vi "SentinelController v33.vi"() -> ()   [LabVIEW 2011] (continued)
                  n321 = property on="System UPH" class="Knob (strict)"("Scale.Minimum"=w3911) -> ()  [unwired: 2 in, 2 out]
                  n322 = property on="H1 UPH" class="Knob (strict)"("Scale.Minimum"=w3911) -> ()  [unwired: 2 in, 2 out]
                  n323 = property on="H2 UPH" class="Knob (strict)"("Scale.Minimum"=w3911) -> ()  [unwired: 2 in, 2 out]
                  n324 = property on="SysUtilMon" class="WFChart (strict)"("History Data"=cluster{dbl, dbl}[] []) -> ()  [unwired: 2 in, 2 out]
                  n325 = local write "H1 alarm"(w3929) -> ()
                  n326 = local write "H2 alarm"(w3929) -> ()
                  n327 = property on="YieldMon" class="WFChart (strict)"("History Data"=cluster{dbl, dbl, dbl, dbl}[] []) -> ()  [unwired: 2 in, 2 out]
                  n328 = local write "YieldMon"(w3906) -> ()
                  n329 = local write "SysUtilMon"(w3905) -> ()
                  n330 = local write "Sys utilization"(0.0) -> ()
                  n331 = local write "H2 alarm 2"(w3929) -> ()
                  n332 = local write "H1 alarm 2"(w3929) -> ()
                  n333 = local write "H2 nominal"(TRUE ("H1 nominal")) -> ()
                  n334 = local write "H1 nominal"(TRUE ("H1 nominal")) -> ()
                  n335 = local read "Lot number"() -> (w3903:string)
                  n336 = local write "Number of text alerts"(0.0 ("Number of Emails Alerts Sent")) -> ()
                  n337 = local write "Number of email alerts"(u32 0 ("Number of Emails Alerts Sent")) -> ()
                  n338 = local write "Tester loop counter hid"(u32 0 ("Tester loop counter")) -> ()
                  n339 = local write "H1 loop counter hid"(u32 0 ("H1 loop counter hid")) -> ()
                  n340 = local write "H2 loop counter hid"(u32 0 ("H2 loop counter hid")) -> ()
                  n341 = local write "H1 Ready with sites"(FALSE ("H1 Ready with sites")) -> ()
                  n342 = local write "H2 Ready with sites"(FALSE ("H1 Ready with sites")) -> ()
                  n343 = local write "GPIB Bus 0 traffic"(w3908) -> ()
                  n344 = local write "Notifications Lot Display"(w3903) -> ()
                  n345 = local write "GPIB bus 1 traffic"(w3908) -> ()
                  n346 = local write "GPIB bus 2 traffic"(w3908) -> ()
                }
              }
              n347 = case shown="True" w3812 {
                frame False {
                }
                frame True {
                  w3888 = FALSE
                  n348 = local read "H1 online"() -> (w3890:bool)
                  n349 = local read "H2 online"() -> (w3889:bool)
                  n350 = Equal?(x=w3890, y=w3888) -> (x = y?=w3892:bool)
                  n351 = Equal?(x=w3888, y=w3889) -> (x = y?=w3891:bool)
                  n352 = Or(x=w3892, y=w3891) -> (x .or. y?=w3887:bool)
                  n353 = case shown="True" w3887 {
                    frame False {
                    }
                    frame True {
                      n354 = local write "Optimize handler speed"(FALSE ("Optimize Handler Speed")) -> ()
                    }
                  }
                }
              }
              n355 = local read "Alert volume"() -> (w3823:u32)
              n356 = Equal To 0?(x=w3823) -> (x = 0?=w3825:bool)
              n357 = case shown="True" w3825 {
                frame False {
                }
                frame True {
                  n358 = local write "Audio On / Off"(FALSE ("Audio On/Off")) -> ()
                }
              }
            }
            n359 = case shown="True" FALSE {
              frame False {
              }
              frame True {
                n360 = while {
                  i -> [w1256]
                  stop <- w1269 stop-if-true
                  # "Play Audio Aert Loop"
                  n361 = local read "Ignore alarms until AFTER this many cycles"() -> (w1261:i32)
                  n362 = local read "H1 Device Count"() -> (w1266:u32)
                  n363 = local read "H2 Device Count"() -> (w1265:u32)
                  n364 = local read "Program Parallelism"() -> (w1263:u32)
                  n365 = local read "Run"() -> (w1258:bool)
                  n366 = local read "POWER"() -> (w1259:bool)
                  n367 = Add(x=w1266, y=w1265) -> (x+y=w1264:u32)
                  n368 = Wait (ms)(milliseconds to wait=u32 100) -> ()  [unwired: 1 out]
                  n369 = Divide(x=w1264, y=w1263) -> (x/y=w1262:dbl)
                  n370 = Greater?(x=w1256, y=50) -> (0:w1254:bool)
                  n371 = Greater?(x=w1262, y=w1261) -> (0:w1260:bool)
                  n372 = Compound Arithmetic op=AND(w1260, w1259, w1258, w1254) -> (w1257:bool)
                  n373 = case shown="True" w1257 {
                    frame False {
                    }
                    frame True {
                      n374 = local read "system statuts hid"() -> (w1273:T8)
                      n375 = case shown="\"H1AH2A\"" w1273 {
                        frame "H1NH2N", Default {
                          n376 = Wait (ms)(milliseconds to wait=u32 50) -> ()  [unwired: 1 out]
                        }
                        frame "H1NH2W" {
                          n377 = flat-sequence {
                            frame #0 {
                              n378 = local read "Audio On / Off"() -> (w1276:bool)
                              n379 = local read "H2 online"() -> (w1275:bool)
                              n380 = And(x=w1275, y=w1276) -> (x .and. y?=w1277:bool)
                              n381 = case shown="True" w1277 {
                                frame False {
                                }
                                frame True {
                                n382 = local read "Run"() -> (w1280:bool)
                                n383 = case shown="True" w1280 {
                                tunnel: [0.001 w1282] -> w1279
                                frame False {
                                }
                                frame True {
                                n384 = local read "Alert volume"() -> (w1282:u32)
                                }
                                }
                                n385 = call "PlayAlarm.vi"("wavefilename"="audio\\4_synth_warning.wav", "alertvolume"=w1279) -> ()  [unwired: 10 in]
                                }
                              }
                            }
                            frame #1 {
                              n386 = local read "Run"() -> (w1283:bool)
                              n387 = case shown="True" w1283 {
                                frame False {
                                }
                                frame True {
                                n388 = Wait (ms)(milliseconds to wait=u32 5000) -> ()  [unwired: 1 out]
                                }
                              }
                            }
                          }
                        }
                        frame "H1NH2A" {
                          n389 = flat-sequence {
                            frame #0 {
                              n390 = local read "Audio On / Off"() -> (w1287:bool)
                              n391 = local read "H2 online"() -> (w1286:bool)
                              n392 = And(x=w1286, y=w1287) -> (x .and. y?=w1285:bool)
                              n393 = case shown="True" w1285 {
                                frame False {
                                }
                                frame True {
                                n394 = local read "Run"() -> (w1290:bool)
                                n395 = case shown="True" w1290 {
                                tunnel: [0.001 w1292] -> w1289
                                frame False {
                                }
                                frame True {
                                n396 = local read "Alert volume"() -> (w1292:u32)
                                }
                                }
                                n397 = call "PlayAlarm.vi"("wavefilename"="audio\\bass_synth_alarm.wav", "alertvolume"=w1289) -> ()  [unwired: 10 in]
                                }
                              }
                            }
                            frame #1 {
                              n398 = local read "Run"() -> (w1293:bool)
                              n399 = case shown="True" w1293 {
                                frame False {
                                n400 = Wait (ms)(milliseconds to wait=u32 50) -> ()  [unwired: 1 out]
                                }
                                frame True {
                                n401 = Wait (ms)(milliseconds to wait=u32 5000) -> ()  [unwired: 1 out]
                                }
                              }
                            }
                          }
                        }
                        frame "H1WH2N" {
                          n402 = flat-sequence {
                            frame #0 {
                              n403 = local read "Audio On / Off"() -> (w1298:bool)
                              n404 = local read "H1 online"() -> (w1297:bool)
                              n405 = And(x=w1297, y=w1298) -> (x .and. y?=w1296:bool)
                              n406 = case shown="True" w1296 {
                                frame False {
                                }
                                frame True {
                                n407 = local read "Run"() -> (w1301:bool)
                                n408 = case shown="True" w1301 {
                                tunnel: [0.001 w1303] -> w1300
                                frame False {
                                }
                                frame True {
                                n409 = local read "Alert volume"() -> (w1303:u32)
                                }
                                }
                                n410 = call "PlayAlarm.vi"("wavefilename"="audio\\4_synth_warning.wav", "alertvolume"=w1300) -> ()  [unwired: 10 in]
                                }
                              }
                            }
                            frame #1 {
                              n411 = local read "Run"() -> (w1304:bool)
                              n412 = case shown="True" w1304 {
                                frame False {
                                n413 = Wait (ms)(milliseconds to wait=u32 50) -> ()  [unwired: 1 out]
                                }
                                frame True {
                                n414 = Wait (ms)(milliseconds to wait=u32 5000) -> ()  [unwired: 1 out]
                                }
                              }
                            }
                          }
                        }
                        frame "H1WH2W" {
                          n415 = flat-sequence {
                            frame #0 {
                              n416 = local read "Audio On / Off"() -> (w1310:bool)
                              n417 = local read "H1 online"() -> (w1307:bool)
                              n418 = local read "H2 online"() -> (w1309:bool)
                              n419 = Compound Arithmetic op=AND(w1307, w1309, w1310) -> (w1308:bool)
                              n420 = case shown="True" w1308 {
                                frame False {
                                }
                                frame True {
                                n421 = local read "Run"() -> (w1313:bool)
                                n422 = case shown="True" w1313 {
                                tunnel: [0.001 w1315] -> w1312
                                frame False {
                                }
                                frame True {
                                n423 = local read "Alert volume"() -> (w1315:u32)
                                }
                                }
                                n424 = call "PlayAlarm.vi"("wavefilename"="audio\\4_synth_warning.wav", "alertvolume"=w1312) -> ()  [unwired: 10 in]
                                }
                              }
                            }
                            frame #1 {
                              n425 = local read "Run"() -> (w1316:bool)
                              n426 = case shown="True" w1316 {
                                frame False {
                                n427 = Wait (ms)(milliseconds to wait=u32 50) -> ()  [unwired: 1 out]
                                }
                                frame True {
                                n428 = Wait (ms)(milliseconds to wait=u32 5000) -> ()  [unwired: 1 out]
                                }
                              }
                            }
                          }
                        }
                        frame "H1WH2A" {
                          n429 = flat-sequence {
                            frame #0 {
                              n430 = local read "Audio On / Off"() -> (w1322:bool)
                              n431 = local read "H1 online"() -> (w1320:bool)
                              n432 = local read "H2 online"() -> (w1321:bool)
                              n433 = Compound Arithmetic op=AND(w1320, w1321, w1322) -> (w1319:bool)
                              n434 = case shown="True" w1319 {
                                frame False {
                                }
                                frame True {
                                n435 = local read "Run"() -> (w1325:bool)
                                n436 = case shown="True" w1325 {
                                tunnel: [0.001 w1327] -> w1324
                                frame False {
                                }
                                frame True {
                                n437 = local read "Alert volume"() -> (w1327:u32)
                                }
                                }
                                n438 = call "PlayAlarm.vi"("wavefilename"="audio\\bass_synth_alarm.wav", "alertvolume"=w1324) -> ()  [unwired: 10 in]
                                }
                              }
                            }
                            frame #1 {
                              n439 = local read "Run"() -> (w1328:bool)
                              n440 = case shown="True" w1328 {
                                frame False {
                                n441 = Wait (ms)(milliseconds to wait=u32 50) -> ()  [unwired: 1 out]
                                }
                                frame True {
                                n442 = Wait (ms)(milliseconds to wait=u32 5000) -> ()  [unwired: 1 out]
                                }
                              }
                            }
                          }
                        }
                        frame "H1AH2N" {
                          n443 = flat-sequence {
                            frame #0 {
                              n444 = local read "Audio On / Off"() -> (w1333:bool)
                              n445 = local read "H1 online"() -> (w1331:bool)
                              n446 = And(x=w1331, y=w1333) -> (x .and. y?=w1332:bool)
                              n447 = case shown="True" w1332 {
                                frame False {
                                }
                                frame True {
                                n448 = local read "Run"() -> (w1336:bool)
                                n449 = case shown="True" w1336 {
                                tunnel: [0.001 w1338] -> w1335
                                frame False {
                                }
                                frame True {
                                n450 = local read "Alert volume"() -> (w1338:u32)
                                }
                                }
                                n451 = call "PlayAlarm.vi"("wavefilename"="audio\\bass_synth_alarm.wav", "alertvolume"=w1335) -> ()  [unwired: 10 in]
                                }
                              }
                            }
                            frame #1 {
                              n452 = local read "Run"() -> (w1339:bool)
                              n453 = case shown="True" w1339 {
                                frame False {
                                n454 = Wait (ms)(milliseconds to wait=u32 50) -> ()  [unwired: 1 out]
                                }
                                frame True {
                                n455 = Wait (ms)(milliseconds to wait=u32 5000) -> ()  [unwired: 1 out]
                                }
                              }
                            }
                          }
                        }
                        frame "H1AH2W" {
                          n456 = flat-sequence {
                            frame #0 {
                              n457 = local read "Audio On / Off"() -> (w1345:bool)
                              n458 = local read "H1 online"() -> (w1343:bool)
                              n459 = local read "H2 online"() -> (w1344:bool)
                              n460 = Compound Arithmetic op=AND(w1343, w1344, w1345) -> (w1342:bool)
                              n461 = case shown="True" w1342 {
                                frame False {
                                }
                                frame True {
                                n462 = local read "Run"() -> (w1348:bool)
                                n463 = case shown="True" w1348 {
                                tunnel: [0.001 w1350] -> w1347
                                frame False {
                                }
                                frame True {
                                n464 = local read "Alert volume"() -> (w1350:u32)
                                }
                                }
                                n465 = call "PlayAlarm.vi"("wavefilename"="audio\\bass_synth_alarm.wav", "alertvolume"=w1347) -> ()  [unwired: 10 in]
                                }
                              }
                            }
                            frame #1 {
                              n466 = local read "Run"() -> (w1351:bool)
                              n467 = case shown="True" w1351 {
                                frame False {
                                n468 = Wait (ms)(milliseconds to wait=u32 50) -> ()  [unwired: 1 out]
                                }
                                frame True {
                                n469 = Wait (ms)(milliseconds to wait=u32 5000) -> ()  [unwired: 1 out]
                                }
                              }
                            }
                          }
                        }
                        frame "H1AH2A" {
                          n470 = flat-sequence {
                            frame #0 {
                              n471 = local read "Audio On / Off"() -> (w1357:bool)
                              n472 = local read "H1 online"() -> (w1355:bool)
                              n473 = local read "H2 online"() -> (w1356:bool)
                              n474 = Compound Arithmetic op=AND(w1355, w1356, w1357) -> (w1354:bool)
                              n475 = case shown="True" w1354 {
                                frame False {
                                }
                                frame True {
                                n476 = local read "Run"() -> (w1360:bool)
                                n477 = case shown="True" w1360 {
                                tunnel: [0.001 w1362] -> w1359
                                frame False {
                                }
                                frame True {
                                n478 = local read "Alert volume"() -> (w1362:u32)
                                }
                                }
                                n479 = call "PlayAlarm.vi"("wavefilename"="audio\\bass_synth_alarm.wav", "alertvolume"=w1359) -> ()  [unwired: 10 in]
                                }
                              }
                            }
                            frame #1 {
                              n480 = local read "Run"() -> (w1363:bool)
                              n481 = case shown="True" w1363 {
                                frame False {
                                n482 = Wait (ms)(milliseconds to wait=u32 50) -> ()  [unwired: 1 out]
                                }
                                frame True {
                                n483 = Wait (ms)(milliseconds to wait=u32 5000) -> ()  [unwired: 1 out]
                                }
                              }
                            }
                          }
                        }
                      }
                    }
                  }
                  n484 = local read "Run"() -> (w1267:bool)
                  n485 = local read "POWER"() -> (w1270:bool)
                  n486 = Not(x=w1270) -> (.not. x?=w1272:bool)
                  n487 = Not(x=w1267) -> (.not. x?=w1271:bool)
                  n488 = Compound Arithmetic op=OR(w1272, w1271) -> (w1269:bool)
                }
              }
            }
            n489 = while {
              shift-right: [w3218] -> _
              shift-left: T8."H1NH2N" ("system statuts") -> [w3208]
              stop <- w3207 continue-if-true
              # "system status state machine:\n- writes data log whenever there is a change (if data loggin enabled)\n- issues email and text alerts is enabled (electronic notification of alarms)"
              n490 = local read "H1 parallelism"() -> (w3214:u32)
              n491 = local read "H1 Device Count"() -> (w3215:u32)
              n492 = local read "H2 Device Count"() -> (w3213:u32)
              n493 = local read "H2 parallelism"() -> (w3212:u32)
              n494 = local read "POWER"() -> (w3207:bool)
              n495 = Divide(x=w3213, y=w3212) -> (x/y=w3209:dbl)
              n496 = Divide(x=w3215, y=w3214) -> (x/y=w3210:dbl)
              n497 = local read "Ignore alarms until AFTER this many cycles"() -> (w3217:i32)
              n498 = Add(x=w3210, y=w3209) -> (x+y=w3211:dbl)
              n499 = Greater?(x=w3211, y=w3217) -> (0:w3216:bool)
              n500 = case shown="True" w3216 {
                tunnel: [w3220 w3223] -> w3218
                tunnel: w3208 -> [w3220 w3221]
                frame False {
                }
                frame True {
                  n501 = flat-sequence {
                    tunnel: [w3224] -> w3222
                    tunnel: w3221 -> [w3224]
                    tunnel: [w3321] -> w3223
                    tunnel: w3222 -> [w3319]
                    frame #0 {
                      # "Determine current state for System Status state-machine"
                      n502 = stacked-sequence {
                        frame #0 {
                          n503 = local read "H1 nominal 2"() -> (w3228:bool)
                          n504 = local read "H2 nominal 2"() -> (w3226:bool)
                          n505 = local read "H1 nominal"() -> (w3229:bool)
                          n506 = local read "H2 nominal"() -> (w3227:bool)
                          n507 = Compound Arithmetic op=AND(w3229, w3228, w3227, w3226) -> (w3225:bool)
                          n508 = case shown="True" w3225 {
                            frame False {
                            }
                            frame True {
                              n509 = local write "system statuts hid"(T8."H1NH2N" ("system statuts")) -> ()
                            }
                          }
                        }
                        frame #1 {
                          n510 = local read "H2 warning 2"() -> (w3233:bool)
                          n511 = local read "H2 warning"() -> (w3234:bool)
                          n512 = local read "H1 nominal 2"() -> (w3235:bool)
                          n513 = local read "H1 nominal"() -> (w3236:bool)
                          n514 = Or(x=w3234, y=w3233) -> (x .or. y?=w3232:bool)
                          n515 = Compound Arithmetic op=AND(w3236, w3235, w3232) -> (w3231:bool)
                          n516 = case shown="False" w3231 {
                            frame False {
                            }
                            frame True {
                              n517 = local write "system statuts hid"(T8."H1NH2W" ("system statuts")) -> ()
                            }
                          }
                        }
                        frame #2 {
                          n518 = local read "H1 nominal 2"() -> (w3243:bool)
                          n519 = local read "H1 nominal"() -> (w3244:bool)
                          n520 = local read "H2 alarm 2"() -> (w3241:bool)
                          n521 = local read "H2 alarm"() -> (w3242:bool)
                          n522 = Or(x=w3242, y=w3241) -> (x .or. y?=w3239:bool)
                          n523 = And(x=w3244, y=w3243) -> (x .and. y?=w3240:bool)
                          n524 = And(x=w3240, y=w3239) -> (x .and. y?=w3238:bool)
                          n525 = case shown="True" w3238 {
                            frame False {
                            }
                            frame True {
                              n526 = local write "system statuts hid"(T8."H1NH2A" ("system statuts")) -> ()
                            }
                          }
                        }
                        frame #3 {
                          n527 = local read "H1 alarm 2"() -> (w3254:bool)
                          n528 = local read "H1 alarm"() -> (w3255:bool)
                          n529 = local read "H2 nominal 2"() -> (w3257:bool)
                          n530 = local read "H1 warning 2"() -> (w3250:bool)
                          n531 = local read "H1 warning"() -> (w3251:bool)
                          n532 = local read "H2 nominal"() -> (w3256:bool)
                          n533 = Not(x=w3255) -> (.not. x?=w3253:bool)
                          n534 = Not(x=w3254) -> (.not. x?=w3252:bool)
                          n535 = Or(x=w3251, y=w3250) -> (x .or. y?=w3248:bool)
                          n536 = And(x=w3253, y=w3252) -> (x .and. y?=w3247:bool)
                          n537 = And(x=w3256, y=w3257) -> (x .and. y?=w3246:bool)
                          n538 = Compound Arithmetic op=AND(w3248, w3247, w3246) -> (w3249:bool)
                          n539 = case shown="True" w3249 {
                            frame False {
                            }
                            frame True {
                              n540 = local write "system statuts hid"(T8."H1WH2N" ("system statuts")) -> ()
                            }
                          }
                        }
                        frame #4 {
                          n541 = local read "H1 alarm 2"() -> (w3269:bool)
                          n542 = local read "H2 alarm 2"() -> (w3274:bool)
                          n543 = local read "H1 alarm"() -> (w3268:bool)
                          n544 = local read "H2 alarm"() -> (w3275:bool)
                          n545 = local read "H1 warning 2"() -> (w3265:bool)
                          n546 = local read "H2 warning 2"() -> (w3266:bool)
                          n547 = local read "H1 warning"() -> (w3264:bool)
                          n548 = local read "H2 warning"() -> (w3267:bool)
                          n549 = Not(x=w3268) -> (.not. x?=w3270:bool)
                          n550 = Not(x=w3269) -> (.not. x?=w3271:bool)
                          n551 = Not(x=w3275) -> (.not. x?=w3273:bool)
                          n552 = Not(x=w3274) -> (.not. x?=w3272:bool)
                          n553 = Or(x=w3264, y=w3265) -> (x .or. y?=w3262:bool)
                          n554 = Or(x=w3267, y=w3266) -> (x .or. y?=w3260:bool)
                          n555 = And(x=w3270, y=w3271) -> (x .and. y?=w3261:bool)
                          n556 = And(x=w3273, y=w3272) -> (x .and. y?=w3259:bool)
                          n557 = Compound Arithmetic op=AND(w3262, w3261, w3260, w3259) -> (w3263:bool)
                          n558 = case shown="True" w3263 {
                            frame False {
                            }
                            frame True {
                              n559 = local write "system statuts hid"(T8."H1WH2W" ("system statuts")) -> ()
                            }
                          }
                        }
                        frame #5 {
                          n560 = local read "H1 alarm 2"() -> (w3282:bool)
                          n561 = local read "H1 alarm"() -> (w3283:bool)
                          n562 = local read "H1 warning 2"() -> (w3285:bool)
                          n563 = local read "H1 warning"() -> (w3286:bool)
                          n564 = local read "H2 alarm 2"() -> (w3287:bool)
                          n565 = local read "H2 alarm"() -> (w3288:bool)
                          n566 = Not(x=w3283) -> (.not. x?=w3281:bool)
                          n567 = Not(x=w3282) -> (.not. x?=w3280:bool)
                          n568 = Or(x=w3286, y=w3285) -> (x .or. y?=w3279:bool)
                          n569 = Or(x=w3288, y=w3287) -> (x .or. y?=w3277:bool)
                          n570 = And(x=w3281, y=w3280) -> (x .and. y?=w3278:bool)
                          n571 = Compound Arithmetic op=AND(w3279, w3278, w3277) -> (w3284:bool)
                          n572 = case shown="True" w3284 {
                            frame False {
                            }
                            frame True {
                              n573 = local write "system statuts hid"(T8."H1WH2A" ("system statuts")) -> ()
                            }
                          }
                        }
                        frame #6 {
                          n574 = local read "H2 nominal 2"() -> (w3295:bool)
                          n575 = local read "H2 nominal"() -> (w3296:bool)
                          n576 = local read "H1 alarm 2"() -> (w3293:bool)
                          n577 = local read "H1 alarm"() -> (w3294:bool)
                          n578 = Or(x=w3294, y=w3293) -> (x .or. y?=w3291:bool)
                          n579 = And(x=w3296, y=w3295) -> (x .and. y?=w3290:bool)
                          n580 = And(x=w3291, y=w3290) -> (x .and. y?=w3292:bool)
                          n581 = case shown="True" w3292 {
                            frame False {
                            }
                            frame True {
                              n582 = local write "system statuts hid"(T8."H1AH2N" ("system statuts")) -> ()
                            }
                          }
                        }
                        frame #7 {
                          n583 = local read "H2 alarm 2"() -> (w3300:bool)
                          n584 = local read "H2 alarm"() -> (w3301:bool)
                          n585 = local read "H2 warning 2"() -> (w3306:bool)
                          n586 = local read "H2 warning"() -> (w3307:bool)
                          n587 = local read "H1 alarm 2"() -> (w3308:bool)
                          n588 = local read "H1 alarm"() -> (w3309:bool)
                          n589 = Not(x=w3301) -> (.not. x?=w3299:bool)
                          n590 = Not(x=w3300) -> (.not. x?=w3298:bool)
                          n591 = Or(x=w3309, y=w3308) -> (x .or. y?=w3304:bool)
                          n592 = Or(x=w3307, y=w3306) -> (x .or. y?=w3303:bool)
                          n593 = And(x=w3299, y=w3298) -> (x .and. y?=w3302:bool)
                          n594 = Compound Arithmetic op=AND(w3304, w3303, w3302) -> (w3305:bool)
                          n595 = case shown="True" w3305 {
                            frame False {
                            }
                            frame True {
                              n596 = local write "system statuts hid"(T8."H1AH2W" ("system statuts")) -> ()
                            }
                          }
                        }
                        frame #8 {
                          n597 = local read "H1 alarm 2"() -> (w3315:bool)
                          n598 = local read "H2 alarm 2"() -> (w3314:bool)
                          n599 = local read "H1 alarm"() -> (w3316:bool)
                          n600 = local read "H2 alarm"() -> (w3313:bool)
                          n601 = Or(x=w3316, y=w3315) -> (x .or. y?=w3311:bool)
                          n602 = Or(x=w3313, y=w3314) -> (x .or. y?=w3312:bool)
                          n603 = And(x=w3311, y=w3312) -> (x .and. y?=w3317:bool)
                          n604 = case shown="True" w3317 {
                            frame False {
                            }
                            frame True {
                              n605 = local write "system statuts hid"(T8."H1AH2A" ("system statuts")) -> ()
                            }
                          }
                        }
                      }
                    }
                    frame #1 {
                      n606 = local read "system statuts hid"() -> (w3321:T8)
                      n607 = Not Equal?(x=w3321, y=w3319) -> (x != y?=w3320:bool)
                      n608 = case shown="True" w3320 {
                        tunnel: w3321 -> [_ w3323]
                        frame False {
                        }
                        frame True {
                          n609 = local read "Enable data logging of all events"() -> (w3322:bool)
                          n610 = case shown="True" w3322 {
                            tunnel: w3323 -> [_ w3324]
                            frame False {
                            }
                            frame True {
                              n611 = stacked-sequence {
                                tunnel: w3324 -> [_ w3327 _ _ _]
                                frame #0 {
                                n612 = local read "Number of data log entries hid"() -> (w3326:u32)
                                n613 = Increment(x=w3326) -> (x+1=w3325:u32)
                                n614 = local write "Number of data log entries hid"(w3325) -> ()
                                }
                                frame #1 {
                                n615 = case shown="\"H1AH2A\"" w3327 {
                                frame "H1NH2N", Default {
                                w3334 = "\r\n"
                                n616 = local read "H1 online"() -> (w3351:bool)
                                n617 = local read "H2 online"() -> (w3352:bool)
                                n618 = local read "Number of data log entries hid"() -> (w3328:u32)
                                n619 = local read "H1 UPH warning limit hid"() -> (w3347:dbl)
                                n620 = local read "H2 UPH warning limit hid"() -> (w3349:dbl)
                                n621 = local read "YieldMon"() -> (w3332:cluster{i32, i32, i32, i32})
                                n622 = local read "H2  low yield warning"() -> (w3348:dbl)
                                n623 = local read "H1 low yield warning"() -> (w3346:dbl)
                                n624 = local read "H1 UPH"() -> (w3340:cluster{u32, u32})
                                n625 = local read "H2 UPH"() -> (w3338:cluster{u32, u32})
                                n626 = local read "YieldMon"() -> (w3330:cluster{i32, i32, i32, i32})
                                n627 = case shown="True" w3351 {
                                tunnel: ["H1 Off-Line" "H1 On-Line"] -> w3353
                                frame False {
                                }
                                frame True {
                                }
                                }
                                n628 = case shown="True" w3352 {
                                tunnel: ["H2 Off-Line" "H2 On-Line"] -> w3362
                                frame False {
                                }
                                frame True {
                                }
                                }
                                n629 = Unbundle(w3332) -> (w3331:i32)  [unwired: 3 out]
                                n630 = Unbundle(w3340) -> (w3339:u32)  [unwired: 1 out]
                                n631 = Unbundle(w3330) -> (w3329:i32)  [unwired: 3 out]
                                n632 = Unbundle(w3338) -> (w3337:u32)  [unwired: 1 out]
                                n633 = local read "Data log path and filename"() -> (w3336:path)
                                n634 = Number To Decimal String(number=w3346) -> (decimal integer string=w3355:string)  [unwired: 1 in]
                                n635 = Number To Decimal String(number=w3331) -> (decimal integer string=w3357:string)  [unwired: 1 in]
                                n636 = Number To Decimal String(number=w3347) -> (decimal integer string=w3359:string)  [unwired: 1 in]
                                n637 = Number To Decimal String(number=w3339) -> (decimal integer string=w3361:string)  [unwired: 1 in]
                                n638 = Number To Decimal String(number=w3348) -> (decimal integer string=w3364:string)  [unwired: 1 in]
                                n639 = Number To Decimal String(number=w3329) -> (decimal integer string=w3366:string)  [unwired: 1 in]
                                n640 = Number To Decimal String(number=w3349) -> (decimal integer string=w3368:string)  [unwired: 1 in]
                                n641 = Number To Decimal String(number=w3337) -> (decimal integer string=w3370:string)  [unwired: 1 in]
                                n642 = Number To Decimal String(number=w3328) -> (decimal integer string=w3333:string)  [unwired: 1 in]
                                n643 = Get Date/Time String(want seconds? (F)=TRUE) -> (date string=w3344:string, time string=w3345:string)  [unwired: 2 in]
                                n644 = Concatenate Strings(w3333, w3334, w3344, "   " ("string"), w3345, w3334, "H1 Nominal, H2 Nominal", w3334, w3353, w3334, "H1 Low Yield Warning Limit: ", w3355, ", H1 yield = ", w3357, w3334, "H1 Low UPH Warning Limit: ", w3359, ", H1 UPH = ", w3361, w3334, w3362, w3334, "H2 Low Yield Warning Limit: ", w3364, ", H2 yield = ", w3366, w3334, "H2 Low UPH Warning Limit: ", w3368, ", H2 UPH = ", w3370, w3334, w3334) -> (w3342:string)
                                n645 = call "SentinelDatalog.vi"("operation (0:open)"=T9."open", "String"=w3342, "data log path"=w3336) -> ()  [unwired: 8 in, 1 out]
                                }
                                frame "H1NH2W" {
                                w3380 = "\r\n"
                                n646 = local read "H1 online"() -> (w3398:bool)
                                n647 = local read "H2 online"() -> (w3399:bool)
                                n648 = local read "H1 UPH warning limit hid"() -> (w3394:dbl)
                                n649 = local read "H2 UPH warning limit hid"() -> (w3396:dbl)
                                n650 = local read "YieldMon"() -> (w3379:cluster{i32, i32, i32, i32})
                                n651 = local read "H2  low yield warning"() -> (w3395:dbl)
                                n652 = local read "H1 low yield warning"() -> (w3393:dbl)
                                n653 = local read "H1 UPH"() -> (w3387:cluster{u32, u32})
                                n654 = local read "H2 UPH"() -> (w3385:cluster{u32, u32})
                                n655 = local read "YieldMon"() -> (w3377:cluster{i32, i32, i32, i32})
                                n656 = local read "Number of data log entries hid"() -> (w3375:u32)
                                n657 = case shown="True" w3398 {
                                tunnel: ["H1 Off-Line" "H1 On-Line"] -> w3400
                                frame False {
                                }
                                frame True {
                                }
                                }
                                n658 = case shown="True" w3399 {
                                tunnel: ["H2 Off-Line" "H2 On-Line"] -> w3409
                                frame False {
                                }
                                frame True {
                                }
                                }
                                n659 = Unbundle(w3377) -> (w3376:i32)  [unwired: 3 out]
                                n660 = Unbundle(w3387) -> (w3386:u32)  [unwired: 1 out]
                                n661 = Unbundle(w3379) -> (w3378:i32)  [unwired: 3 out]
                                n662 = Unbundle(w3385) -> (w3384:u32)  [unwired: 1 out]
                                n663 = Number To Decimal String(number=w3393) -> (decimal integer string=w3402:string)  [unwired: 1 in]
                                n664 = Number To Decimal String(number=w3376) -> (decimal integer string=w3404:string)  [unwired: 1 in]
                                n665 = Number To Decimal String(number=w3394) -> (decimal integer string=w3406:string)  [unwired: 1 in]
                                n666 = Number To Decimal String(number=w3386) -> (decimal integer string=w3408:string)  [unwired: 1 in]
                                n667 = Number To Decimal String(number=w3395) -> (decimal integer string=w3411:string)  [unwired: 1 in]
                                n668 = Number To Decimal String(number=w3378) -> (decimal integer string=w3413:string)  [unwired: 1 in]
                                n669 = Number To Decimal String(number=w3396) -> (decimal integer string=w3415:string)  [unwired: 1 in]
                                n670 = Number To Decimal String(number=w3384) -> (decimal integer string=w3417:string)  [unwired: 1 in]
                                n671 = Number To Decimal String(number=w3375) -> (decimal integer string=w3381:string)  [unwired: 1 in]
                                n672 = local read "Data log path and filename"() -> (w3383:path)
                                n673 = Get Date/Time String(want seconds? (F)=TRUE) -> (date string=w3391:string, time string=w3392:string)  [unwired: 2 in]
                                n674 = Concatenate Strings(w3381, w3380, w3391, "   " ("string"), w3392, w3380, "H1 Nominal, H2 Warning", w3380, w3400, w3380, "H1 Low Yield Warning Limit: ", w3402, ", H1 yield = ", w3404, w3380, "H1 Low UPH Warning Limit: ", w3406, ", H1 UPH = ", w3408, w3380, w3409, w3380, "H2 Low Yield Warning Limit: ", w3411, ", H2 yield = ", w3413, w3380, "H2 Low UPH Warning Limit: ", w3415, ", H2 UPH = ", w3417, w3380, w3380) -> (w3389:string)
                                n675 = call "SentinelDatalog.vi"("operation (0:open)"=T9."open", "String"=w3389, "data log path"=w3383) -> ()  [unwired: 8 in, 1 out]
                                }
                                frame "H1NH2A" {
                                w3428 = "\r\n"
                                n676 = local read "H1 online"() -> (w3445:bool)
                                n677 = local read "H2 online"() -> (w3446:bool)
                                n678 = local read "Number of data log entries hid"() -> (w3422:u32)
                                n679 = local read "H1 UPH warning limit hid"() -> (w3441:dbl)
                                n680 = local read "H1 low yield warning"() -> (w3440:dbl)
                                n681 = local read "H2 UPH alarm limit hid"() -> (w3443:dbl)
                                n682 = local read "YieldMon"() -> (w3426:cluster{i32, i32, i32, i32})
                                n683 = local read "H1 UPH"() -> (w3434:cluster{u32, u32})
                                n684 = local read "H2 low yield alarm"() -> (w3442:dbl)
                                n685 = local read "H2 UPH"() -> (w3433:cluster{u32, u32})
                                n686 = local read "YieldMon"() -> (w3424:cluster{i32, i32, i32, i32})
                                n687 = case shown="True" w3445 {
                                tunnel: ["H1 Off-Line" "H1 On-Line"] -> w3447
                                frame False {
                                }
                                frame True {
                                }
                                }
                                n688 = case shown="True" w3446 {
                                tunnel: ["H2 Off-Line" "H2 On-Line"] -> w3456
                                frame False {
                                }
                                frame True {
                                }
                                }
                                n689 = Number To Decimal String(number=w3422) -> (decimal integer string=w3427:string)  [unwired: 1 in]
                                n690 = Unbundle(w3426) -> (w3425:i32)  [unwired: 3 out]
                                n691 = Unbundle(w3434) -> (w3431:u32)  [unwired: 1 out]
                                n692 = Unbundle(w3424) -> (w3423:i32)  [unwired: 3 out]
                                n693 = Unbundle(w3433) -> (w3432:u32)  [unwired: 1 out]
                                n694 = Number To Decimal String(number=w3440) -> (decimal integer string=w3449:string)  [unwired: 1 in]
                                n695 = Number To Decimal String(number=w3425) -> (decimal integer string=w3451:string)  [unwired: 1 in]
                                n696 = Number To Decimal String(number=w3441) -> (decimal integer string=w3453:string)  [unwired: 1 in]
                                n697 = Number To Decimal String(number=w3431) -> (decimal integer string=w3455:string)  [unwired: 1 in]
                                n698 = Number To Decimal String(number=w3442) -> (decimal integer string=w3458:string)  [unwired: 1 in]
                                n699 = Number To Decimal String(number=w3423) -> (decimal integer string=w3460:string)  [unwired: 1 in]
                                n700 = Number To Decimal String(number=w3443) -> (decimal integer string=w3462:string)  [unwired: 1 in]
                                n701 = Number To Decimal String(number=w3432) -> (decimal integer string=w3464:string)  [unwired: 1 in]
                                n702 = local read "Data log path and filename"() -> (w3430:path)
                                n703 = Get Date/Time String(want seconds? (F)=TRUE) -> (date string=w3438:string, time string=w3439:string)  [unwired: 2 in]
                                n704 = Concatenate Strings(w3427, w3428, w3438, "   " ("string"), w3439, w3428, "H1 Nominal, H2 Alarming", w3428, w3447, w3428, "H1 Low Yield Warning Limit: ", w3449, ", H1 yield = ", w3451, w3428, "H1 Low UPH Warning Limit: ", w3453, ", H1 UPH = ", w3455, w3428, w3456, w3428, "H2 Low Yield Alarm Limit: ", w3458, ", H2 yield = ", w3460, w3428, "H2 Low UPH Alarm Limit: ", w3462, ", H2 UPH = ", w3464, w3428, w3428) -> (w3436:string)
                                n705 = call "SentinelDatalog.vi"("operation (0:open)"=T9."open", "String"=w3436, "data log path"=w3430) -> ()  [unwired: 8 in, 1 out]
                                }
                                frame "H1WH2N" {
                                w3475 = "\r\n"
                                n706 = local read "H1 online"() -> (w3493:bool)
                                n707 = local read "H2 online"() -> (w3494:bool)
                                n708 = local read "H1 UPH warning limit hid"() -> (w3489:dbl)
                                n709 = local read "H2 UPH warning limit hid"() -> (w3491:dbl)
                                n710 = local read "H2  low yield warning"() -> (w3490:dbl)
                                n711 = local read "H1 low yield warning"() -> (w3488:dbl)
                                n712 = local read "H1 UPH"() -> (w3481:cluster{u32, u32})
                                n713 = local read "H2 UPH"() -> (w3480:cluster{u32, u32})
                                n714 = local read "YieldMon"() -> (w3473:cluster{i32, i32, i32, i32})
                                n715 = local read "YieldMon"() -> (w3471:cluster{i32, i32, i32, i32})
                                n716 = local read "Number of data log entries hid"() -> (w3469:u32)
                                n717 = case shown="True" w3493 {
                                tunnel: ["H1 Off-Line" "H1 On-Line"] -> w3482
                                frame False {
                                }
                                frame True {
                                }
                                }
                                n718 = case shown="True" w3494 {
                                tunnel: ["H2 Off-Line" "H2 On-Line"] -> w3503
                                frame False {
                                }
                                frame True {
                                }
                                }
                                n719 = Unbundle(w3473) -> (w3472:i32)  [unwired: 3 out]
                                n720 = Unbundle(w3481) -> (w3478:u32)  [unwired: 1 out]
                                n721 = Unbundle(w3471) -> (w3470:i32)  [unwired: 3 out]
                                n722 = Unbundle(w3480) -> (w3479:u32)  [unwired: 1 out]
                                n723 = Number To Decimal String(number=w3488) -> (decimal integer string=w3496:string)  [unwired: 1 in]
                                n724 = Number To Decimal String(number=w3472) -> (decimal integer string=w3498:string)  [unwired: 1 in]
                                n725 = Number To Decimal String(number=w3489) -> (decimal integer string=w3500:string)  [unwired: 1 in]
                                n726 = Number To Decimal String(number=w3478) -> (decimal integer string=w3502:string)  [unwired: 1 in]
                                n727 = Number To Decimal String(number=w3490) -> (decimal integer string=w3505:string)  [unwired: 1 in]
                                n728 = Number To Decimal String(number=w3470) -> (decimal integer string=w3507:string)  [unwired: 1 in]
                                n729 = Number To Decimal String(number=w3491) -> (decimal integer string=w3509:string)  [unwired: 1 in]
                                n730 = Number To Decimal String(number=w3479) -> (decimal integer string=w3511:string)  [unwired: 1 in]
                                n731 = local read "Data log path and filename"() -> (w3477:path)
                                n732 = Number To Decimal String(number=w3469) -> (decimal integer string=w3474:string)  [unwired: 1 in]
                                n733 = Get Date/Time String(want seconds? (F)=TRUE) -> (date string=w3486:string, time string=w3487:string)  [unwired: 2 in]
                                n734 = Concatenate Strings(w3474, w3475, w3486, "   " ("string"), w3487, w3475, "H1 Warning, H2 Nominal", w3475, w3482, w3475, "H1 Low Yield Warning Limit: ", w3496, ", H1 yield = ", w3498, w3475, "H1 Low UPH Warning Limit: ", w3500, ", H1 UPH = ", w3502, w3475, w3503, w3475, "H2 Low Yield Warning Limit: ", w3505, ", H2 yield = ", w3507, w3475, "H2 Low UPH Warning Limit: ", w3509, ", H2 UPH = ", w3511, w3475, w3475) -> (w3484:string)
                                n735 = call "SentinelDatalog.vi"("operation (0:open)"=T9."open", "String"=w3484, "data log path"=w3477) -> ()  [unwired: 8 in, 1 out]
                                }
                                frame "H1WH2W" {
                                w3521 = "\r\n"
                                w3529 = "\r\n"
                                n736 = local read "H1 online"() -> (w3540:bool)
                                n737 = local read "H2 online"() -> (w3541:bool)
                                n738 = local read "H1 UPH warning limit hid"() -> (w3536:dbl)
                                n739 = local read "H2 UPH warning limit hid"() -> (w3538:dbl)
                                n740 = local read "H2  low yield warning"() -> (w3537:dbl)
                                n741 = local read "H1 low yield warning"() -> (w3535:dbl)
                                n742 = local read "H1 UPH"() -> (w3528:cluster{u32, u32})
                                n743 = local read "H2 UPH"() -> (w3527:cluster{u32, u32})
                                n744 = local read "YieldMon"() -> (w3520:cluster{i32, i32, i32, i32})
                                n745 = local read "YieldMon"() -> (w3518:cluster{i32, i32, i32, i32})
                                n746 = case shown="True" w3540 {
                                tunnel: ["H1 Off-Line" "H1 On-Line"] -> w3542
                                frame False {
                                }
                                frame True {
                                }
                                }
                                n747 = case shown="True" w3541 {
                                tunnel: ["H2 Off-Line" "H2 On-Line"] -> w3551
                                frame False {
                                }
                                frame True {
                                }
                                }
                                n748 = local read "Number of data log entries hid"() -> (w3516:u32)
                                n749 = Unbundle(w3520) -> (w3519:i32)  [unwired: 3 out]
                                n750 = Unbundle(w3528) -> (w3526:u32)  [unwired: 1 out]
                                n751 = Unbundle(w3518) -> (w3517:i32)  [unwired: 3 out]
                                n752 = Unbundle(w3527) -> (w3525:u32)  [unwired: 1 out]
                                n753 = Number To Decimal String(number=w3535) -> (decimal integer string=w3544:string)  [unwired: 1 in]
                                n754 = Number To Decimal String(number=w3519) -> (decimal integer string=w3546:string)  [unwired: 1 in]
                                n755 = Number To Decimal String(number=w3536) -> (decimal integer string=w3548:string)  [unwired: 1 in]
                                n756 = Number To Decimal String(number=w3526) -> (decimal integer string=w3550:string)  [unwired: 1 in]
                                n757 = Number To Decimal String(number=w3537) -> (decimal integer string=w3553:string)  [unwired: 1 in]
                                n758 = Number To Decimal String(number=w3517) -> (decimal integer string=w3555:string)  [unwired: 1 in]
                                n759 = Number To Decimal String(number=w3538) -> (decimal integer string=w3557:string)  [unwired: 1 in]
                                n760 = Number To Decimal String(number=w3525) -> (decimal integer string=w3559:string)  [unwired: 1 in]
                                n761 = local read "Data log path and filename"() -> (w3524:path)
                                n762 = Get Date/Time String(want seconds? (F)=TRUE) -> (date string=w3533:string, time string=w3534:string)  [unwired: 2 in]
                                n763 = Number To Decimal String(number=w3516) -> (decimal integer string=w3522:string)  [unwired: 1 in]
                                n764 = Concatenate Strings(w3522, w3521, w3533, "   " ("string"), w3534, w3521, "H1 Warning, H2 Warning", w3521, w3542, w3521, "H1 Low Yield Warning Limit: ", w3544, ", H1 yield = ", w3546, w3529, "H1 Low UPH Warning Limit: ", w3548, ", H1 UPH = ", w3550, w3529, w3551, w3529, "H2 Low Yield Warning Limit: ", w3553, ", H2 yield = ", w3555, w3529, "H2 Low UPH Warning Limit: ", w3557, ", H2 UPH = ", w3559, w3529, w3529) -> (w3531:string)
                                n765 = call "SentinelDatalog.vi"("operation (0:open)"=T9."open", "String"=w3531, "data log path"=w3524) -> ()  [unwired: 8 in, 1 out]
                                }
                                frame "H1WH2A" {
                                w3570 = "\r\n"
                                n766 = local read "H1 online"() -> (w3587:bool)
                                n767 = local read "H2 online"() -> (w3588:bool)
                                n768 = local read "H1 UPH warning limit hid"() -> (w3583:dbl)
                                n769 = local read "H1 low yield warning"() -> (w3582:dbl)
                                n770 = local read "H2 UPH alarm limit hid"() -> (w3585:dbl)
                                n771 = local read "H1 UPH"() -> (w3576:cluster{u32, u32})
                                n772 = local read "H2 low yield alarm"() -> (w3584:dbl)
                                n773 = local read "H2 UPH"() -> (w3575:cluster{u32, u32})
                                n774 = local read "YieldMon"() -> (w3566:cluster{i32, i32, i32, i32})
                                n775 = local read "YieldMon"() -> (w3568:cluster{i32, i32, i32, i32})
                                n776 = local read "Number of data log entries hid"() -> (w3564:u32)
                                n777 = case shown="True" w3587 {
                                tunnel: ["H1 Off-Line" "H1 On-Line"] -> w3589
                                frame False {
                                }
                                frame True {
                                }
                                }
                                n778 = case shown="True" w3588 {
                                tunnel: ["H2 Off-Line" "H2 On-Line"] -> w3598
                                frame False {
                                }
                                frame True {
                                }
                                }
                                n779 = Unbundle(w3566) -> (w3565:i32)  [unwired: 3 out]
                                n780 = Unbundle(w3576) -> (w3574:u32)  [unwired: 1 out]
                                n781 = Unbundle(w3568) -> (w3567:i32)  [unwired: 3 out]
                                n782 = Unbundle(w3575) -> (w3573:u32)  [unwired: 1 out]
                                n783 = Number To Decimal String(number=w3582) -> (decimal integer string=w3591:string)  [unwired: 1 in]
                                n784 = Number To Decimal String(number=w3565) -> (decimal integer string=w3593:string)  [unwired: 1 in]
                                n785 = Number To Decimal String(number=w3583) -> (decimal integer string=w3595:string)  [unwired: 1 in]
                                n786 = Number To Decimal String(number=w3574) -> (decimal integer string=w3597:string)  [unwired: 1 in]
                                n787 = Number To Decimal String(number=w3584) -> (decimal integer string=w3600:string)  [unwired: 1 in]
                                n788 = Number To Decimal String(number=w3567) -> (decimal integer string=w3602:string)  [unwired: 1 in]
                                n789 = Number To Decimal String(number=w3585) -> (decimal integer string=w3604:string)  [unwired: 1 in]
                                n790 = Number To Decimal String(number=w3573) -> (decimal integer string=w3606:string)  [unwired: 1 in]
                                n791 = local read "Data log path and filename"() -> (w3572:path)
                                n792 = Get Date/Time String(want seconds? (F)=TRUE) -> (date string=w3580:string, time string=w3581:string)  [unwired: 2 in]
                                n793 = Number To Decimal String(number=w3564) -> (decimal integer string=w3569:string)  [unwired: 1 in]
                                n794 = Concatenate Strings(w3569, w3570, w3580, "   " ("string"), w3581, w3570, "H1 Warning, H2 Alarming", w3570, w3589, w3570, "H1 Low Yield Warning Limit: ", w3591, ", H1 yield = ", w3593, w3570, "H1 Low UPH Warning Limit: ", w3595, ", H1 UPH = ", w3597, w3570, w3598, w3570, "H2 Low Yield Alarm Limit: ", w3600, ", H2 yield = ", w3602, w3570, "H2 Low UPH Alarm Limit: ", w3604, ", H2 UPH = ", w3606, w3570, w3570) -> (w3578:string)
                                n795 = call "SentinelDatalog.vi"("operation (0:open)"=T9."open", "String"=w3578, "data log path"=w3572) -> ()  [unwired: 8 in, 1 out]
                                }
                                frame "H1AH2N" {
                                w3617 = "\r\n"
                                n796 = local read "H1 online"() -> (w3634:bool)
                                n797 = local read "H2 online"() -> (w3635:bool)
                                n798 = local read "H2 UPH warning limit hid"() -> (w3632:dbl)
                                n799 = local read "H2  low yield warning"() -> (w3631:dbl)
                                n800 = local read "H1 UPH alarm limit hid"() -> (w3630:dbl)
                                n801 = local read "H1 low yield alarm"() -> (w3629:dbl)
                                n802 = local read "H1 UPH"() -> (w3623:cluster{u32, u32})
                                n803 = local read "H2 UPH"() -> (w3622:cluster{u32, u32})
                                n804 = local read "YieldMon"() -> (w3615:cluster{i32, i32, i32, i32})
                                n805 = local read "YieldMon"() -> (w3613:cluster{i32, i32, i32, i32})
                                n806 = case shown="True" w3634 {
                                tunnel: ["H1 Off-Line" "H1 On-Line"] -> w3636
                                frame False {
                                }
                                frame True {
                                }
                                }
                                n807 = case shown="False" w3635 {
                                tunnel: ["H2 Off-Line" "H2 On-Line"] -> w3645
                                frame False {
                                }
                                frame True {
                                }
                                }
